vi "Device Manager Check if Running.vi"(7 "Notifier Name":string) -> (8 "Running?":bool)   [LabVIEW 2020]
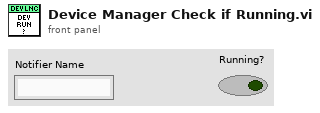
[diagram p1: front panel]
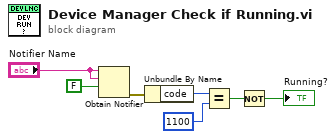
[diagram p0: block diagram]
diagram:
  n1 = Obtain Notifier(name (unnamed)="Notifier Name", notification data type="Notifier Name", create if not found? (T)=FALSE) -> (error out=w6:errorcluster)  [unwired: 1 in, 2 out]
  n2 = Unbundle By Name(w6) -> ("code"=w5:i32)
  n3 = Equal?(x=w5, y=1100) -> (x = y?=w2:bool)
  n4 = Not(x=w2) -> (.not. x?=→"Running?":bool)
